vi "Enemy (sub vi).vi"(8 "Direct in":i32, 9 "position in":i32[](array[numeric]), 11 "boarder":i32[][](array[numeric])=[[0, 0, 18, 0], [0, 1, 18, 1], [0, 2, 18, 2], [0, 3, 18, 3], [0, 4, 18, 4], [0, 5, 18, 5], [0, 6, 18, 6], [0, 7, 18, 7], [0, 8, 18, 8], [0, 9, 18, 9], [0, 10, 18, 10], [0, 11, 18, 11], [0, 12, 18, 12], [0, 13, 18, 13], [0, 14, 18, 14], [0, 15, 18, 15], [0, 16, 18, 16], [0, 17, 18, 17], [0, 18, 18, 18], [18, 0, 19, 19], [18, 1, 0, 0], [18, 2, 0, 0], [18, 3, 0, 0], [18, 4, 0, 0], [18, 5, 0, 0], [18, 6, 0, 0], [18, 7, 0, 0], [18, 8, 0, 0], [18, 9, 0, 0], [18, 10, 0, 0], [18, 11, 0, 0], [18, 12, 0, 0], [18, 13, 0, 0], [18, 14, 0, 0], [18, 15, 0, 0], [18, 16, 0, 0], [18, 17, 0, 0], [18, 18, 0, 0], [0, 0, 0, 0], [1, 0, 0, 0], [2, 0, 0, 0], [3, 0, 0, 0], [4, 0, 0, 0], [5, 0, 0, 0], [6, 0, 0, 0], [7, 0, 0, 0], [8, 0, 0, 0], [9, 0, 0, 0], [10, 0, 0, 0], [11, 0, 0, 0], [12, 0, 0, 0], [13, 0, 0, 0], [14, 0, 0, 0], [15, 0, 0, 0], [16, 0, 0, 0], [17, 0, 0, 0], [18, 0, 0, 0], [0, 18, 0, 0], [1, 18, 0, 0], [2, 18, 0, 0], [3, 18, 0, 0], [4, 18, 0, 0], [5, 18, 0, 0], [6, 18, 0, 0], [7, 18, 0, 0], [8, 18, 0, 0], [9, 18, 0, 0], [10, 18, 0, 0], [11, 18, 0, 0], [12, 18, 0, 0], [13, 18, 0, 0], [14, 18, 0, 0], [15, 18, 0, 0], [16, 18, 0, 0], [17, 18, 0, 0], [18, 18, 0, 0], [2, 2, 0, 0], [2, 3, 0, 0], [2, 4, 0, 0], [2, 5, 0, 0], [2, 6, 0, 0], [3, 6, 0, 0], [4, 6, 0, 0], [4, 7, 0, 0], [4, 8, 0, 0], [3, 8, 0, 0], [2, 8, 0, 0], [4, 2, 0, 0], [4, 3, 0, 0], [4, 4, 0, 0], [5, 2, 0, 0], [6, 2, 0, 0], [7, 2, 0, 0], [8, 2, 0, 0], [10, 1, 0, 0], [10, 2, 0, 0], [12, 2, 0, 0], [12, 3, 0, 0], [13, 3, 0, 0], [14, 3, 0, 0], [14, 1, 0, 0], [16, 2, 0, 0], [16, 3, 0, 0], [16, 4, 0, 0], [16, 5, 0, 0], [16, 6, 0, 0], [16, 7, 0, 0], [14, 5, 0, 0], [15, 5, 0, 0], [6, 4, 0, 0], [7, 4, 0, 0], [8, 4, 0, 0], [9, 4, 0, 0], [10, 4, 0, 0], [12, 5, 0, 0], [12, 6, 0, 0], [12, 7, 0, 0], [6, 6, 0, 0], [7, 6, 0, 0], [8, 6, 0, 0], [7, 7, 0, 0], [7, 8, 0, 0], [7, 9, 0, 0], [7, 10, 0, 0], [7, 11, 0, 0], [6, 12, 0, 0], [7, 12, 0, 0], [8, 12, 0, 0], [10, 6, 0, 0], [10, 7, 0, 0], [10, 8, 0, 0], [10, 9, 0, 0], [10, 10, 0, 0], [10, 11, 0, 0], [10, 12, 0, 0], [11, 9, 0, 0], [12, 9, 0, 0], [14, 7, 0, 0], [14, 8, 0, 0], [14, 9, 0, 0], [14, 10, 0, 0], [14, 11, 0, 0], [15, 9, 0, 0], [16, 9, 0, 0], [2, 10, 0, 0], [3, 10, 0, 0], [4, 10, 0, 0], [4, 11, 0, 0], [4, 12, 0, 0], [3, 12, 0, 0], [2, 12, 0, 0], [2, 13, 0, 0], [2, 14, 0, 0], [2, 15, 0, 0], [2, 16, 0, 0], [4, 14, 0, 0], [4, 15, 0, 0], [4, 16, 0, 0], [5, 16, 0, 0], [6, 16, 0, 0], [7, 16, 0, 0], [8, 16, 0, 0], [6, 14, 0, 0], [7, 14, 0, 0], [8, 14, 0, 0], [9, 14, 0, 0], [10, 14, 0, 0], [10, 16, 0, 0], [10, 17, 0, 0], [14, 17, 0, 0], [12, 15, 0, 0], [13, 15, 0, 0], [14, 15, 0, 0], [12, 16, 0, 0], [12, 11, 0, 0], [12, 12, 0, 0], [12, 13, 0, 0], [14, 13, 0, 0], [15, 13, 0, 0], [16, 11, 0, 0], [16, 12, 0, 0], [16, 13, 0, 0], [16, 14, 0, 0], [16, 15, 0, 0], [16, 16, 0, 0]]) -> (0 "Direct out":i32, 3 "position out":i32[](array[numeric]))   [LabVIEW 2014]
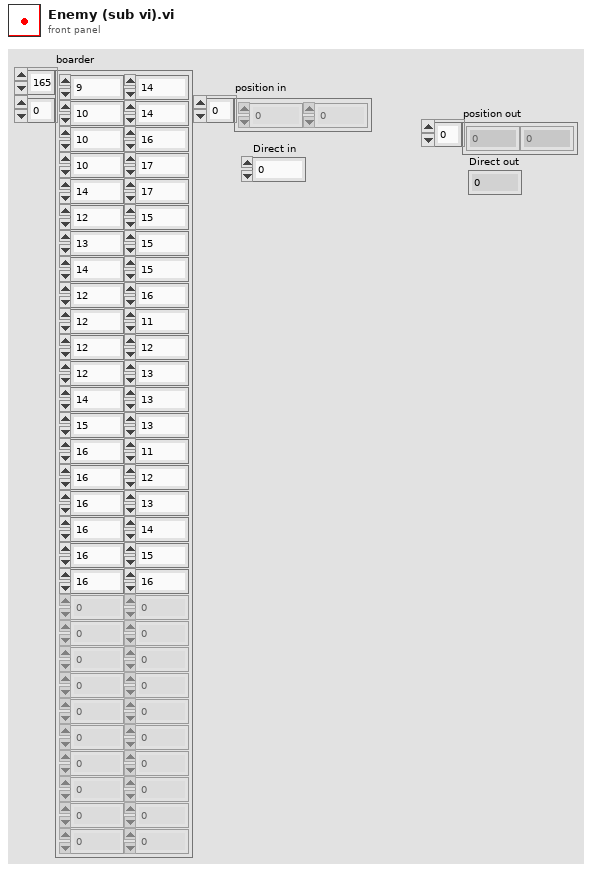
[diagram p1: front panel]
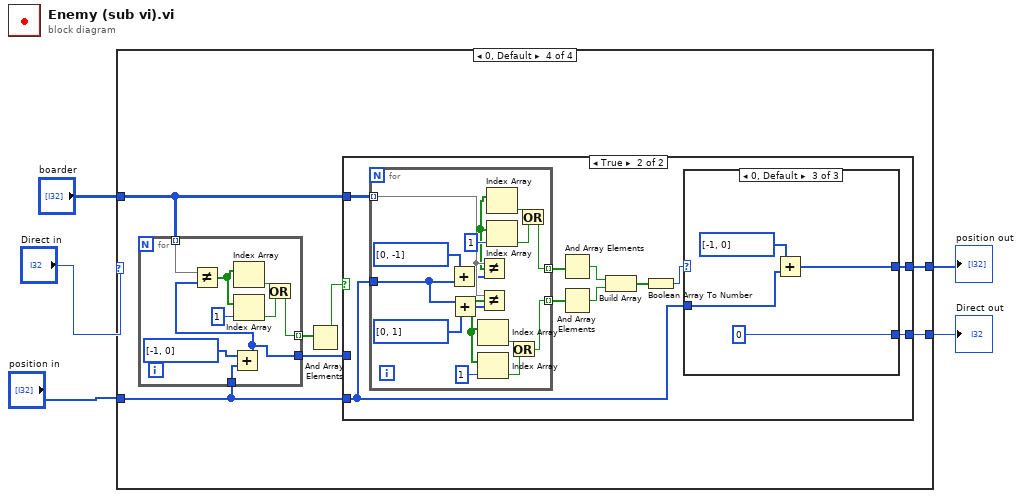
[diagram p0: block diagram]
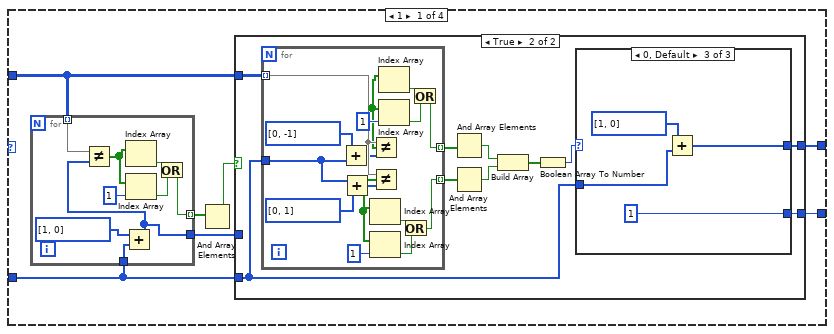
[diagram p2: hidden frame]
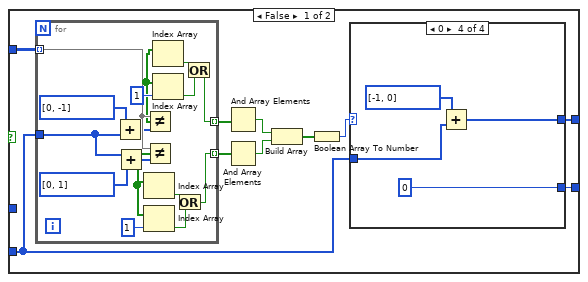
[diagram p3: hidden frame]
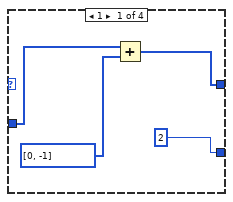
[diagram p4: hidden frame]
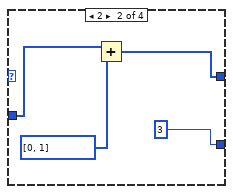
[diagram p5: hidden frame]
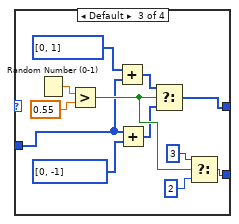
[diagram p6: hidden frame]
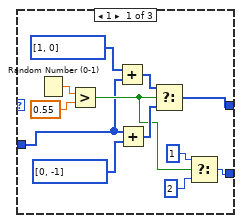
[diagram p7: hidden frame]
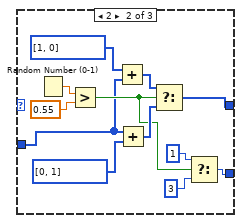
[diagram p8: hidden frame]
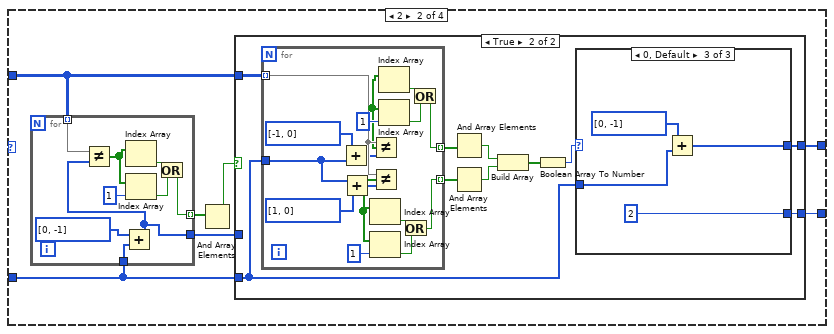
[diagram p9: hidden frame]
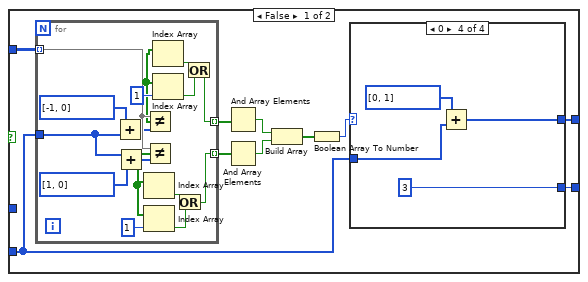
[diagram p10: hidden frame]
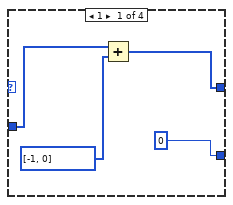
[diagram p11: hidden frame]
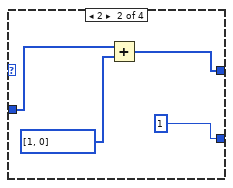
[diagram p12: hidden frame]
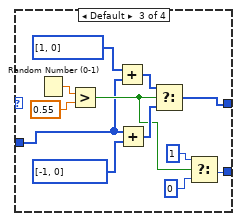
[diagram p13: hidden frame]
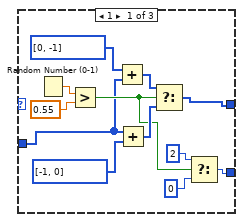
[diagram p14: hidden frame]
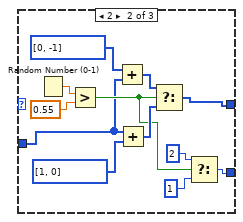
[diagram p15: hidden frame]
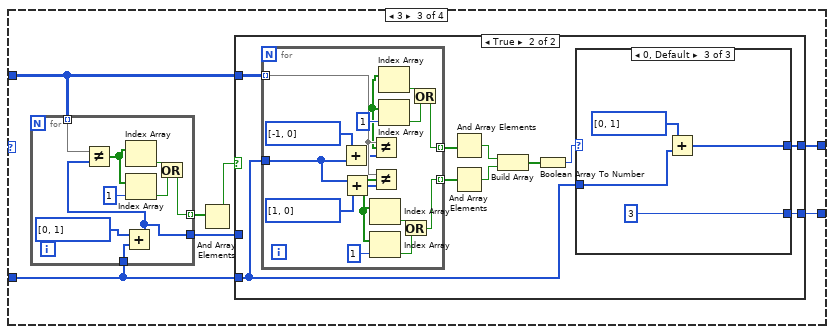
[diagram p16: hidden frame]
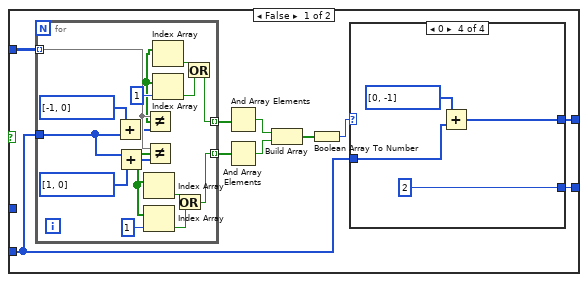
[diagram p17: hidden frame]
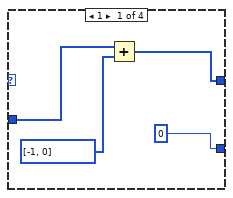
[diagram p18: hidden frame]
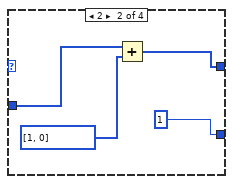
[diagram p19: hidden frame]
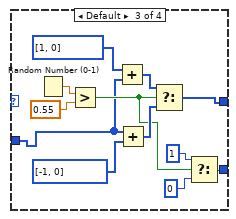
[diagram p20: hidden frame]
diagram:
  n1 = case shown="0, Default" "Direct in" {
    tunnel: "position in" -> [w8 w128 w248 w368]
    tunnel: "boarder" -> [w7 w127 w247 w367]
    tunnel: [w12 w132 w252 w372] -> w3
    tunnel: [w11 w131 w251 w371] -> w2
    frame 1 {
      n2 = for {
        tunnel: w8 -> [w124]
        tunnel: w7 -> [w123] mode=indexing
        tunnel: [w118] -> w10 mode=indexing
        tunnel: [w117] -> w6
        n3 = Add(x=i32[] [1, 0], y=w124) -> (x+y=w117:i32[])
        n4 = Not Equal?(x=w123, y=w117) -> (x != y?=w119:bool[])
        n5 = Index Array(array=w119) -> (element=w120:bool)  [unwired: 1 in]
        n6 = Index Array(array=w119, index=1) -> (element=w121:bool)
        n7 = Or(x=w120, y=w121) -> (x .or. y?=w118:bool)
      }
      n8 = And Array Elements(Boolean array=w10) -> (logical AND=w9:bool)
      n9 = case shown="True" w9 {
        tunnel: w7 -> [w22 w72]
        tunnel: w8 -> [w15 w65]
        tunnel: [w14 w64] -> w12
        tunnel: [w13 w63] -> w11
        tunnel: w6 -> [_ _]
        frame False {
          n10 = for {
            tunnel: w15 -> [w60]
            tunnel: w22 -> [w59] mode=indexing
            tunnel: [w48] -> w21 mode=indexing
            tunnel: [w47] -> w20 mode=indexing
            n11 = Add(x=i32[] [0, -1], y=w60) -> (x+y=w58:i32[])
            n12 = Add(x=w60, y=i32[] [0, 1]) -> (x+y=w57:i32[])
            n13 = Not Equal?(x=w59, y=w58) -> (x != y?=w50:bool[])
            n14 = Not Equal?(x=w59, y=w57) -> (x != y?=w49:bool[])
            n15 = Index Array(array=w49) -> (element=w51:bool)  [unwired: 1 in]
            n16 = Index Array(array=w49, index=1) -> (element=w52:bool)
            n17 = Index Array(array=w50) -> (element=w54:bool)  [unwired: 1 in]
            n18 = Index Array(array=w50, index=1) -> (element=w55:bool)
            n19 = Or(x=w51, y=w52) -> (x .or. y?=w47:bool)
            n20 = Or(x=w54, y=w55) -> (x .or. y?=w48:bool)
          }
          n21 = And Array Elements(Boolean array=w21) -> (logical AND=w19:bool)
          n22 = And Array Elements(Boolean array=w20) -> (logical AND=w18:bool)
          n23 = Build Array(w19, w18) -> (w17:bool[])
          n24 = Boolean Array To Number(Boolean array=w17) -> (number=w16:u32)
          n25 = case shown="0" w16 {
            tunnel: w15 -> [w24 w27 w33 w45]
            tunnel: [w23 w29 w32 w44] -> w14
            tunnel: [2 3 w31 0] -> w13
            frame 1 {
              n26 = Add(x=w24, y=i32[] [0, -1]) -> (x+y=w23:i32[])
            }
            frame 2 {
              n27 = Add(x=w27, y=i32[] [0, 1]) -> (x+y=w29:i32[])
            }
            frame Default {
              n28 = Random Number (0-1)() -> (number: 0 to 1=w34:dbl)
              n29 = Greater?(x=w34, y=0.55) -> (0:w40:bool)
              n30 = Add(x=i32[] [0, 1], y=w33) -> (x+y=w38:i32[])
              n31 = Add(x=w33, y=i32[] [0, -1]) -> (x+y=w39:i32[])
              n32 = Select(t=w38, s=w40, f=w39) -> (s? t:f=w32:i32[])
              n33 = Select(t=3, s=w40, f=2) -> (s? t:f=w31:i32)
            }
            frame 0 {
              n34 = Add(x=i32[] [-1, 0], y=w45) -> (x+y=w44:i32[])
            }
          }
        }
        frame True {
          n35 = for {
            tunnel: w65 -> [w114]
            tunnel: w72 -> [w113] mode=indexing
            tunnel: [w102] -> w71 mode=indexing
            tunnel: [w101] -> w70 mode=indexing
            n36 = Add(x=i32[] [0, -1], y=w114) -> (x+y=w112:i32[])
            n37 = Add(x=w114, y=i32[] [0, 1]) -> (x+y=w111:i32[])
            n38 = Not Equal?(x=w113, y=w112) -> (x != y?=w104:bool[])
            n39 = Not Equal?(x=w113, y=w111) -> (x != y?=w103:bool[])
            n40 = Index Array(array=w103) -> (element=w105:bool)  [unwired: 1 in]
            n41 = Index Array(array=w103, index=1) -> (element=w106:bool)
            n42 = Index Array(array=w104) -> (element=w108:bool)  [unwired: 1 in]
            n43 = Index Array(array=w104, index=1) -> (element=w109:bool)
            n44 = Or(x=w105, y=w106) -> (x .or. y?=w101:bool)
            n45 = Or(x=w108, y=w109) -> (x .or. y?=w102:bool)
          }
          n46 = And Array Elements(Boolean array=w71) -> (logical AND=w69:bool)
          n47 = And Array Elements(Boolean array=w70) -> (logical AND=w68:bool)
          n48 = Build Array(w69, w68) -> (w67:bool[])
          n49 = Boolean Array To Number(Boolean array=w67) -> (number=w66:u32)
          n50 = case shown="0, Default" w66 {
            tunnel: w65 -> [w73 w85 w99]
            tunnel: [w75 w87 w98] -> w64
            tunnel: [w74 w86 1] -> w63
            frame 1 {
              n51 = Random Number (0-1)() -> (number: 0 to 1=w84:dbl)
              n52 = Greater?(x=w84, y=0.55) -> (0:w78:bool)
              n53 = Add(x=i32[] [1, 0], y=w73) -> (x+y=w80:i32[])
              n54 = Add(x=w73, y=i32[] [0, -1]) -> (x+y=w79:i32[])
              n55 = Select(t=w80, s=w78, f=w79) -> (s? t:f=w75:i32[])
              n56 = Select(t=1, s=w78, f=2) -> (s? t:f=w74:i32)
            }
            frame 2 {
              n57 = Random Number (0-1)() -> (number: 0 to 1=w96:dbl)
              n58 = Greater?(x=w96, y=0.55) -> (0:w90:bool)
              n59 = Add(x=i32[] [1, 0], y=w85) -> (x+y=w92:i32[])
              n60 = Add(x=w85, y=i32[] [0, 1]) -> (x+y=w91:i32[])
              n61 = Select(t=w92, s=w90, f=w91) -> (s? t:f=w87:i32[])
              n62 = Select(t=1, s=w90, f=3) -> (s? t:f=w86:i32)
            }
            frame 0, Default {
              n63 = Add(x=i32[] [1, 0], y=w99) -> (x+y=w98:i32[])
            }
          }
        }
      }
    }
    frame 2 {
      n64 = for {
        tunnel: w128 -> [w244]
        tunnel: w127 -> [w243] mode=indexing
        tunnel: [w238] -> w130 mode=indexing
        tunnel: [w237] -> w126
        n65 = Add(x=i32[] [0, -1], y=w244) -> (x+y=w237:i32[])
        n66 = Not Equal?(x=w243, y=w237) -> (x != y?=w239:bool[])
        n67 = Index Array(array=w239) -> (element=w240:bool)  [unwired: 1 in]
        n68 = Index Array(array=w239, index=1) -> (element=w241:bool)
        n69 = Or(x=w240, y=w241) -> (x .or. y?=w238:bool)
      }
      n70 = And Array Elements(Boolean array=w130) -> (logical AND=w129:bool)
      n71 = case shown="True" w129 {
        tunnel: w127 -> [w142 w192]
        tunnel: w128 -> [w135 w185]
        tunnel: [w134 w184] -> w132
        tunnel: [w133 w183] -> w131
        tunnel: w126 -> [_ _]
        frame False {
          n72 = for {
            tunnel: w135 -> [w180]
            tunnel: w142 -> [w179] mode=indexing
            tunnel: [w168] -> w141 mode=indexing
            tunnel: [w167] -> w140 mode=indexing
            n73 = Add(x=i32[] [-1, 0], y=w180) -> (x+y=w178:i32[])
            n74 = Add(x=w180, y=i32[] [1, 0]) -> (x+y=w177:i32[])
            n75 = Not Equal?(x=w179, y=w178) -> (x != y?=w170:bool[])
            n76 = Not Equal?(x=w179, y=w177) -> (x != y?=w169:bool[])
            n77 = Index Array(array=w169) -> (element=w171:bool)  [unwired: 1 in]
            n78 = Index Array(array=w169, index=1) -> (element=w172:bool)
            n79 = Index Array(array=w170) -> (element=w174:bool)  [unwired: 1 in]
            n80 = Index Array(array=w170, index=1) -> (element=w175:bool)
            n81 = Or(x=w171, y=w172) -> (x .or. y?=w167:bool)
            n82 = Or(x=w174, y=w175) -> (x .or. y?=w168:bool)
          }
          n83 = And Array Elements(Boolean array=w141) -> (logical AND=w139:bool)
          n84 = And Array Elements(Boolean array=w140) -> (logical AND=w138:bool)
          n85 = Build Array(w139, w138) -> (w137:bool[])
          n86 = Boolean Array To Number(Boolean array=w137) -> (number=w136:u32)
          n87 = case shown="0" w136 {
            tunnel: w135 -> [w143 w149 w153 w165]
            tunnel: [w145 w147 w152 w164] -> w134
            tunnel: [0 1 w151 3] -> w133
            frame 1 {
              n88 = Add(x=w143, y=i32[] [-1, 0]) -> (x+y=w145:i32[])
            }
            frame 2 {
              n89 = Add(x=w149, y=i32[] [1, 0]) -> (x+y=w147:i32[])
            }
            frame Default {
              n90 = Random Number (0-1)() -> (number: 0 to 1=w162:dbl)
              n91 = Greater?(x=w162, y=0.55) -> (0:w156:bool)
              n92 = Add(x=i32[] [1, 0], y=w153) -> (x+y=w158:i32[])
              n93 = Add(x=w153, y=i32[] [-1, 0]) -> (x+y=w157:i32[])
              n94 = Select(t=w158, s=w156, f=w157) -> (s? t:f=w152:i32[])
              n95 = Select(t=1, s=w156, f=0) -> (s? t:f=w151:i32)
            }
            frame 0 {
              n96 = Add(x=i32[] [0, 1], y=w165) -> (x+y=w164:i32[])
            }
          }
        }
        frame True {
          n97 = for {
            tunnel: w185 -> [w234]
            tunnel: w192 -> [w233] mode=indexing
            tunnel: [w222] -> w191 mode=indexing
            tunnel: [w221] -> w190 mode=indexing
            n98 = Add(x=i32[] [-1, 0], y=w234) -> (x+y=w232:i32[])
            n99 = Add(x=w234, y=i32[] [1, 0]) -> (x+y=w231:i32[])
            n100 = Not Equal?(x=w233, y=w232) -> (x != y?=w224:bool[])
            n101 = Not Equal?(x=w233, y=w231) -> (x != y?=w223:bool[])
            n102 = Index Array(array=w223) -> (element=w225:bool)  [unwired: 1 in]
            n103 = Index Array(array=w223, index=1) -> (element=w226:bool)
            n104 = Index Array(array=w224) -> (element=w228:bool)  [unwired: 1 in]
            n105 = Index Array(array=w224, index=1) -> (element=w229:bool)
            n106 = Or(x=w225, y=w226) -> (x .or. y?=w221:bool)
            n107 = Or(x=w228, y=w229) -> (x .or. y?=w222:bool)
          }
          n108 = And Array Elements(Boolean array=w191) -> (logical AND=w189:bool)
          n109 = And Array Elements(Boolean array=w190) -> (logical AND=w188:bool)
          n110 = Build Array(w189, w188) -> (w187:bool[])
          n111 = Boolean Array To Number(Boolean array=w187) -> (number=w186:u32)
          n112 = case shown="0, Default" w186 {
            tunnel: w185 -> [w193 w205 w219]
            tunnel: [w195 w207 w218] -> w184
            tunnel: [w194 w206 2] -> w183
            frame 1 {
              n113 = Random Number (0-1)() -> (number: 0 to 1=w204:dbl)
              n114 = Greater?(x=w204, y=0.55) -> (0:w198:bool)
              n115 = Add(x=i32[] [0, -1], y=w193) -> (x+y=w200:i32[])
              n116 = Add(x=w193, y=i32[] [-1, 0]) -> (x+y=w199:i32[])
              n117 = Select(t=w200, s=w198, f=w199) -> (s? t:f=w195:i32[])
              n118 = Select(t=2, s=w198, f=0) -> (s? t:f=w194:i32)
            }
            frame 2 {
              n119 = Random Number (0-1)() -> (number: 0 to 1=w216:dbl)
              n120 = Greater?(x=w216, y=0.55) -> (0:w210:bool)
              n121 = Add(x=i32[] [0, -1], y=w205) -> (x+y=w212:i32[])
              n122 = Add(x=w205, y=i32[] [1, 0]) -> (x+y=w211:i32[])
              n123 = Select(t=w212, s=w210, f=w211) -> (s? t:f=w207:i32[])
              n124 = Select(t=2, s=w210, f=1) -> (s? t:f=w206:i32)
            }
            frame 0, Default {
              n125 = Add(x=i32[] [0, -1], y=w219) -> (x+y=w218:i32[])
            }
          }
        }
      }
    }
    frame 3 {
      n126 = for {
        tunnel: w248 -> [w364]
        tunnel: w247 -> [w363] mode=indexing
        tunnel: [w358] -> w250 mode=indexing
        tunnel: [w357] -> w246
        n127 = Add(x=i32[] [0, 1], y=w364) -> (x+y=w357:i32[])
        n128 = Not Equal?(x=w363, y=w357) -> (x != y?=w359:bool[])
        n129 = Index Array(array=w359) -> (element=w360:bool)  [unwired: 1 in]
        n130 = Index Array(array=w359, index=1) -> (element=w361:bool)
        n131 = Or(x=w360, y=w361) -> (x .or. y?=w358:bool)
      }
      n132 = And Array Elements(Boolean array=w250) -> (logical AND=w249:bool)
      n133 = case shown="True" w249 {
        tunnel: w247 -> [w262 w312]
        tunnel: w248 -> [w255 w305]
        tunnel: [w254 w304] -> w252
        tunnel: [w253 w303] -> w251
        tunnel: w246 -> [_ _]
        frame False {
          n134 = for {
            tunnel: w255 -> [w300]
            tunnel: w262 -> [w299] mode=indexing
            tunnel: [w288] -> w261 mode=indexing
            tunnel: [w287] -> w260 mode=indexing
            n135 = Add(x=i32[] [-1, 0], y=w300) -> (x+y=w298:i32[])
            n136 = Add(x=w300, y=i32[] [1, 0]) -> (x+y=w297:i32[])
            n137 = Not Equal?(x=w299, y=w298) -> (x != y?=w290:bool[])
            n138 = Not Equal?(x=w299, y=w297) -> (x != y?=w289:bool[])
            n139 = Index Array(array=w289) -> (element=w291:bool)  [unwired: 1 in]
            n140 = Index Array(array=w289, index=1) -> (element=w292:bool)
            n141 = Index Array(array=w290) -> (element=w294:bool)  [unwired: 1 in]
            n142 = Index Array(array=w290, index=1) -> (element=w295:bool)
            n143 = Or(x=w291, y=w292) -> (x .or. y?=w287:bool)
            n144 = Or(x=w294, y=w295) -> (x .or. y?=w288:bool)
          }
          n145 = And Array Elements(Boolean array=w261) -> (logical AND=w259:bool)
          n146 = And Array Elements(Boolean array=w260) -> (logical AND=w258:bool)
          n147 = Build Array(w259, w258) -> (w257:bool[])
          n148 = Boolean Array To Number(Boolean array=w257) -> (number=w256:u32)
          n149 = case shown="0" w256 {
            tunnel: w255 -> [w265 w269 w273 w285]
            tunnel: [w264 w267 w271 w284] -> w254
            tunnel: [0 1 w272 2] -> w253
            frame 1 {
              n150 = Add(x=w265, y=i32[] [-1, 0]) -> (x+y=w264:i32[])
            }
            frame 2 {
              n151 = Add(x=w269, y=i32[] [1, 0]) -> (x+y=w267:i32[])
            }
            frame Default {
              n152 = Random Number (0-1)() -> (number: 0 to 1=w282:dbl)
              n153 = Greater?(x=w282, y=0.55) -> (0:w276:bool)
              n154 = Add(x=i32[] [1, 0], y=w273) -> (x+y=w278:i32[])
              n155 = Add(x=w273, y=i32[] [-1, 0]) -> (x+y=w277:i32[])
              n156 = Select(t=w278, s=w276, f=w277) -> (s? t:f=w271:i32[])
              n157 = Select(t=1, s=w276, f=0) -> (s? t:f=w272:i32)
            }
            frame 0 {
              n158 = Add(x=i32[] [0, -1], y=w285) -> (x+y=w284:i32[])
            }
          }
        }
        frame True {
          n159 = for {
            tunnel: w305 -> [w354]
            tunnel: w312 -> [w353] mode=indexing
            tunnel: [w342] -> w311 mode=indexing
            tunnel: [w341] -> w310 mode=indexing
            n160 = Add(x=i32[] [-1, 0], y=w354) -> (x+y=w352:i32[])
            n161 = Add(x=w354, y=i32[] [1, 0]) -> (x+y=w351:i32[])
            n162 = Not Equal?(x=w353, y=w352) -> (x != y?=w344:bool[])
            n163 = Not Equal?(x=w353, y=w351) -> (x != y?=w343:bool[])
            n164 = Index Array(array=w343) -> (element=w345:bool)  [unwired: 1 in]
            n165 = Index Array(array=w343, index=1) -> (element=w346:bool)
            n166 = Index Array(array=w344) -> (element=w348:bool)  [unwired: 1 in]
            n167 = Index Array(array=w344, index=1) -> (element=w349:bool)
            n168 = Or(x=w345, y=w346) -> (x .or. y?=w341:bool)
            n169 = Or(x=w348, y=w349) -> (x .or. y?=w342:bool)
          }
          n170 = And Array Elements(Boolean array=w311) -> (logical AND=w309:bool)
          n171 = And Array Elements(Boolean array=w310) -> (logical AND=w308:bool)
          n172 = Build Array(w309, w308) -> (w307:bool[])
          n173 = Boolean Array To Number(Boolean array=w307) -> (number=w306:u32)
          n174 = case shown="0, Default" w306 {
            tunnel: w305 -> [w313 w325 w339]
            tunnel: [w315 w327 w338] -> w304
            tunnel: [w314 w326 3] -> w303
            frame 1 {
              n175 = Random Number (0-1)() -> (number: 0 to 1=w324:dbl)
              n176 = Greater?(x=w324, y=0.55) -> (0:w318:bool)
              n177 = Add(x=i32[] [0, 1], y=w313) -> (x+y=w320:i32[])
              n178 = Add(x=w313, y=i32[] [-1, 0]) -> (x+y=w319:i32[])
              n179 = Select(t=w320, s=w318, f=w319) -> (s? t:f=w315:i32[])
              n180 = Select(t=3, s=w318, f=0) -> (s? t:f=w314:i32)
            }
            frame 2 {
              n181 = Random Number (0-1)() -> (number: 0 to 1=w336:dbl)
              n182 = Greater?(x=w336, y=0.55) -> (0:w330:bool)
              n183 = Add(x=i32[] [0, 1], y=w325) -> (x+y=w332:i32[])
              n184 = Add(x=w325, y=i32[] [1, 0]) -> (x+y=w331:i32[])
              n185 = Select(t=w332, s=w330, f=w331) -> (s? t:f=w327:i32[])
              n186 = Select(t=3, s=w330, f=1) -> (s? t:f=w326:i32)
            }
            frame 0, Default {
              n187 = Add(x=i32[] [0, 1], y=w339) -> (x+y=w338:i32[])
            }
          }
        }
      }
    }
    frame 0, Default {
      n188 = for {
        tunnel: w368 -> [w484]
        tunnel: w367 -> [w483] mode=indexing
        tunnel: [w478] -> w370 mode=indexing
        tunnel: [w477] -> w366
        n189 = Add(x=i32[] [-1, 0], y=w484) -> (x+y=w477:i32[])
        n190 = Not Equal?(x=w483, y=w477) -> (x != y?=w479:bool[])
        n191 = Index Array(array=w479) -> (element=w480:bool)  [unwired: 1 in]
        n192 = Index Array(array=w479, index=1) -> (element=w481:bool)
        n193 = Or(x=w480, y=w481) -> (x .or. y?=w478:bool)
      }
      n194 = And Array Elements(Boolean array=w370) -> (logical AND=w369:bool)
      n195 = case shown="True" w369 {
        tunnel: w367 -> [w382 w432]
        tunnel: w368 -> [w375 w425]
        tunnel: [w374 w424] -> w372
        tunnel: [w373 w423] -> w371
        tunnel: w366 -> [_ _]
        frame False {
          n196 = for {
            tunnel: w375 -> [w420]
            tunnel: w382 -> [w419] mode=indexing
            tunnel: [w408] -> w381 mode=indexing
            tunnel: [w407] -> w380 mode=indexing
            n197 = Add(x=i32[] [0, -1], y=w420) -> (x+y=w418:i32[])
            n198 = Add(x=w420, y=i32[] [0, 1]) -> (x+y=w417:i32[])
            n199 = Not Equal?(x=w419, y=w418) -> (x != y?=w410:bool[])
            n200 = Not Equal?(x=w419, y=w417) -> (x != y?=w409:bool[])
            n201 = Index Array(array=w409) -> (element=w411:bool)  [unwired: 1 in]
            n202 = Index Array(array=w409, index=1) -> (element=w412:bool)
            n203 = Index Array(array=w410) -> (element=w414:bool)  [unwired: 1 in]
            n204 = Index Array(array=w410, index=1) -> (element=w415:bool)
            n205 = Or(x=w411, y=w412) -> (x .or. y?=w407:bool)
            n206 = Or(x=w414, y=w415) -> (x .or. y?=w408:bool)
          }
          n207 = And Array Elements(Boolean array=w381) -> (logical AND=w379:bool)
          n208 = And Array Elements(Boolean array=w380) -> (logical AND=w378:bool)
          n209 = Build Array(w379, w378) -> (w377:bool[])
          n210 = Boolean Array To Number(Boolean array=w377) -> (number=w376:u32)
          n211 = case shown="0" w376 {
            tunnel: w375 -> [w384 w387 w393 w405]
            tunnel: [w383 w389 w392 w404] -> w374
            tunnel: [2 3 w391 1] -> w373
            frame 1 {
              n212 = Add(x=w384, y=i32[] [0, -1]) -> (x+y=w383:i32[])
            }
            frame 2 {
              n213 = Add(x=w387, y=i32[] [0, 1]) -> (x+y=w389:i32[])
            }
            frame Default {
              n214 = Random Number (0-1)() -> (number: 0 to 1=w402:dbl)
              n215 = Greater?(x=w402, y=0.55) -> (0:w396:bool)
              n216 = Add(x=i32[] [0, 1], y=w393) -> (x+y=w398:i32[])
              n217 = Add(x=w393, y=i32[] [0, -1]) -> (x+y=w397:i32[])
              n218 = Select(t=w398, s=w396, f=w397) -> (s? t:f=w392:i32[])
              n219 = Select(t=3, s=w396, f=2) -> (s? t:f=w391:i32)
            }
            frame 0 {
              n220 = Add(x=i32[] [1, 0], y=w405) -> (x+y=w404:i32[])
            }
          }
        }
        frame True {
          n221 = for {
            tunnel: w425 -> [w474]
            tunnel: w432 -> [w473] mode=indexing
            tunnel: [w462] -> w431 mode=indexing
            tunnel: [w461] -> w430 mode=indexing
            n222 = Add(x=i32[] [0, -1], y=w474) -> (x+y=w472:i32[])
            n223 = Add(x=w474, y=i32[] [0, 1]) -> (x+y=w471:i32[])
            n224 = Not Equal?(x=w473, y=w472) -> (x != y?=w464:bool[])
            n225 = Not Equal?(x=w473, y=w471) -> (x != y?=w463:bool[])
            n226 = Index Array(array=w463) -> (element=w465:bool)  [unwired: 1 in]
            n227 = Index Array(array=w463, index=1) -> (element=w466:bool)
            n228 = Index Array(array=w464) -> (element=w468:bool)  [unwired: 1 in]
            n229 = Index Array(array=w464, index=1) -> (element=w469:bool)
            n230 = Or(x=w465, y=w466) -> (x .or. y?=w461:bool)
            n231 = Or(x=w468, y=w469) -> (x .or. y?=w462:bool)
          }
          n232 = And Array Elements(Boolean array=w431) -> (logical AND=w429:bool)
          n233 = And Array Elements(Boolean array=w430) -> (logical AND=w428:bool)
          n234 = Build Array(w429, w428) -> (w427:bool[])
          n235 = Boolean Array To Number(Boolean array=w427) -> (number=w426:u32)
          n236 = case shown="0, Default" w426 {
            tunnel: w425 -> [w433 w445 w459]
            tunnel: [w435 w447 w458] -> w424
            tunnel: [w434 w446 0] -> w423
            frame 1 {
              n237 = Random Number (0-1)() -> (number: 0 to 1=w444:dbl)
              n238 = Greater?(x=w444, y=0.55) -> (0:w438:bool)
              n239 = Add(x=i32[] [-1, 0], y=w433) -> (x+y=w440:i32[])
              n240 = Add(x=w433, y=i32[] [0, -1]) -> (x+y=w439:i32[])
              n241 = Select(t=w440, s=w438, f=w439) -> (s? t:f=w435:i32[])
              n242 = Select(t=0, s=w438, f=2) -> (s? t:f=w434:i32)
            }
            frame 2 {
              n243 = Random Number (0-1)() -> (number: 0 to 1=w456:dbl)
              n244 = Greater?(x=w456, y=0.55) -> (0:w450:bool)
              n245 = Add(x=i32[] [-1, 0], y=w445) -> (x+y=w452:i32[])
              n246 = Add(x=w445, y=i32[] [0, 1]) -> (x+y=w451:i32[])
              n247 = Select(t=w452, s=w450, f=w451) -> (s? t:f=w447:i32[])
              n248 = Select(t=0, s=w450, f=3) -> (s? t:f=w446:i32)
            }
            frame 0, Default {
              n249 = Add(x=i32[] [-1, 0], y=w459) -> (x+y=w458:i32[])
            }
          }
        }
      }
    }
  }
  "position out" <- w3
  "Direct out" <- w2
